vi "Delta_w.vi"(9 "O_(L-1)":dbl, 10 "Delta_L":dbl, 11 "etta":dbl) -> (2 "Delta_w":dbl)   [LabVIEW 2014]
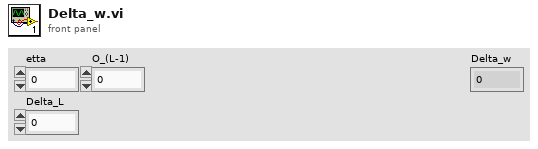
[diagram p1: front panel]
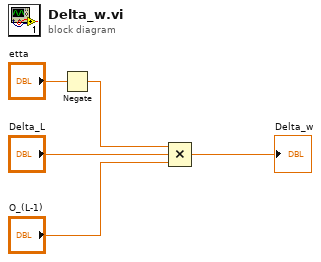
[diagram p0: block diagram]
diagram:
  n1 = Negate(x="etta") -> (-x=w2:dbl)
  n2 = Compound Arithmetic op=MULTIPLY(w2, "Delta_L", "O_(L-1)") -> (→"Delta_w":dbl)
